vi "Write File.vi"(7 "Section":string, 8 "error in (no error)":errorcluster, 10 "Parameters":refnum<class "Parameter.lvclass">[](array[class]), 11 "Parameter INI File in":refnum<class "Parameter INI File.lvclass">) -> (0 "error out":errorcluster, 3 "Parameter INI File out":refnum<class "Parameter INI File.lvclass">)   [LabVIEW 2019, in "CD Parameter Manager API.lvlib" / "Parameter INI File.lvclass"]
uses:
  Parameter INI File.lvclass
  Parameter Class/Parameter.lvclass
  Parameter INI File.lvclass/Parameter INI File.ctl
  Double Parameter Class/Double Parameter.lvclass
  C:/Repositories/CSD_Custom_Device/CSD_Custom_Device/Source/Libraries/CD Parameter Manager API/Parameter Class/Parameter.lvclass
  Parameter Class/Parameter.lvclass/Parameter.ctl
  Double Parameter Class/Double Parameter.lvclass/Double Parameter.ctl
  Boolean Parameter Class/Boolean Parameter.lvclass
  Boolean Parameter Class/Boolean Parameter.lvclass/Boolean Parameter.ctl
  I32 Parameter Class/I32 Parameter.lvclass
  I32 Parameter Class/I32 Parameter.lvclass/I32 Parameter.ctl
  String Parameter Class/String Parameter.lvclass
  String Parameter Class/String Parameter.lvclass/String Parameter.ctl
  File Path Parameter Class/File Path Parameter.lvclass
  File Path Parameter Class/File Path Parameter.lvclass/File Path Parameter.ctl
  Parameter Class/Member Accessors/Read Control label.vi
  Double Parameter Class/Member Accessors/Read Value.vi
  Boolean Parameter Class/Member Accessors/Read Value.vi
  I32 Parameter Class/Member Accessors/Read Value.vi
  String Parameter Class/Member Accessors/Read Value.vi
  File Path Parameter Class/Member Accessors/Read Value.vi
  <vilib>/Utility/config.llb/Write Key (Double).vi
  <vilib>/Utility/config.llb/Write Key (Boolean).vi
  <vilib>/Utility/config.llb/Write Key (I32).vi
  <vilib>/Utility/config.llb/Write Key (String).vi
  <vilib>/Utility/config.llb/Write Key (Path).vi
  <vilib>/Utility/error.llb/Error Cluster From Error Code.vi
  <vilib>/ErrorRing/Error Ring.xnode
  <vilib>/Utility/config.llb/NI_LVConfig.lvlib
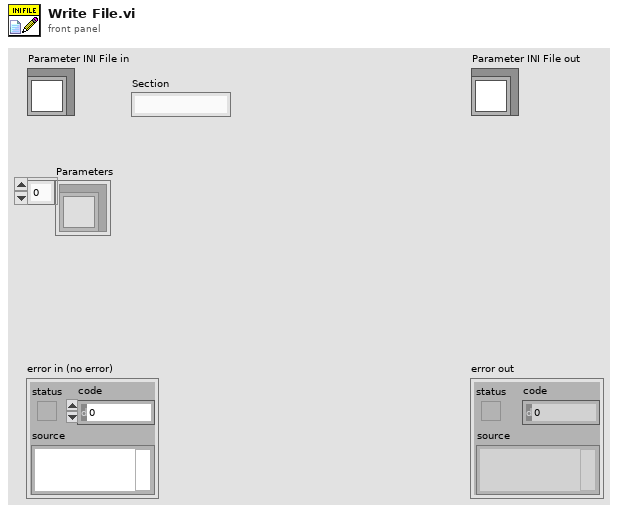
[diagram p1: front panel]
types:
  T1 = typedef "NI_LVConfig.lvlib/Config Data RefNum.ctl" = refnum<k1>
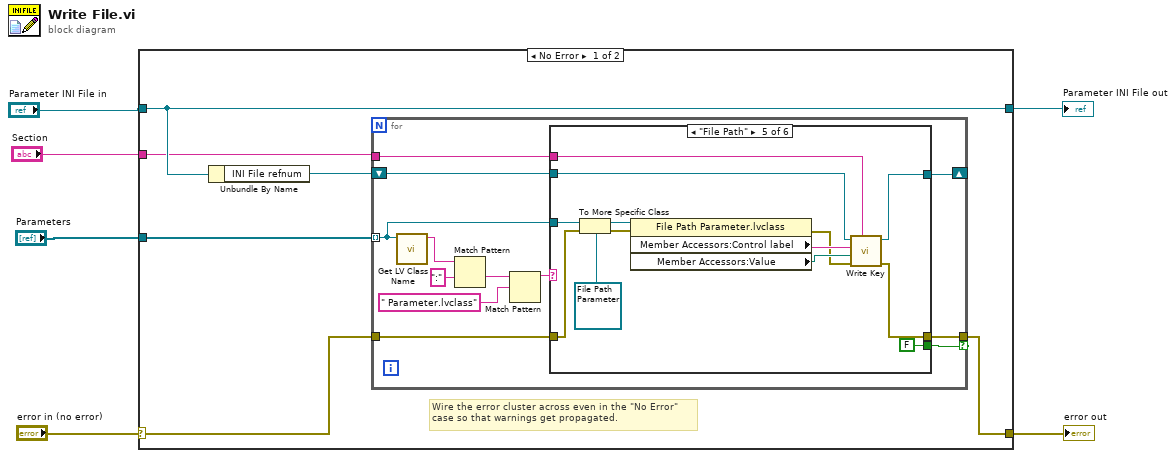
[diagram p0: block diagram]
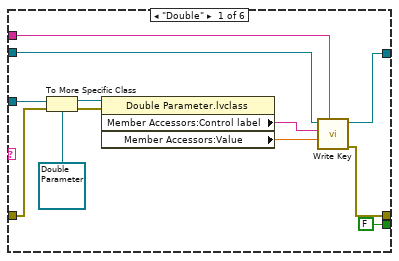
[diagram p2: hidden frame]
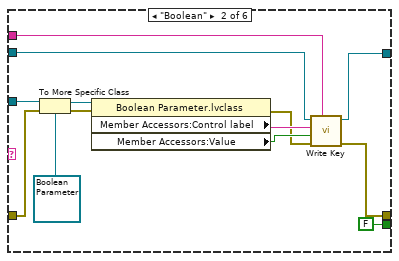
[diagram p3: hidden frame]
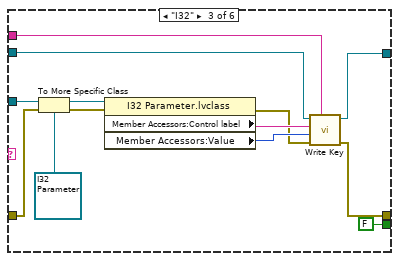
[diagram p4: hidden frame]
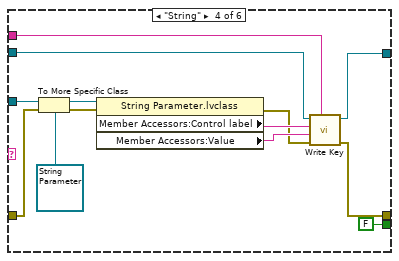
[diagram p5: hidden frame]
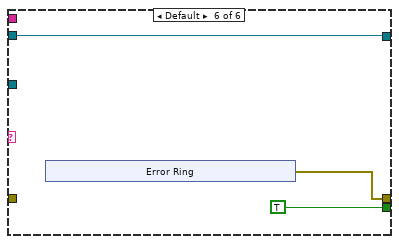
[diagram p6: hidden frame]
diagram:
  n1 = case shown="No Error" "error in (no error)" {
    selector: "error in (no error)" -> [w12 w98]
    tunnel: [w11 w98] -> w3
    tunnel: [w10 w97] -> w4
    tunnel: "Parameter INI File in" -> [w10 w97]
    tunnel: "Parameters" -> [w8 _]
    tunnel: "Section" -> [w7 _]
    frame No Error {
      # "Wire the error cluster across even in the \"No Error\"\ncase so that warnings get propagated."
      n2 = Unbundle By Name(w10) -> ("INI File refnum"=w9:T1)
      n3 = for {
        tunnel: w12 -> [w19]
        tunnel: [w14] -> w11 if=w15
        tunnel: w8 -> [w17] mode=indexing
        tunnel: w7 -> [w16]
        shift-right: [w13] -> _
        shift-left: w9 -> [w18]
        n4 = call <vilib>:"Get LV Class Name.vi"("object"=w17) -> ("class name"=w21:string)  [unwired: 9 in, 1 out]
        n5 = Match Pattern(string=w21, regular expression=":") -> (after substring=w23:string)  [unwired: 1 in, 3 out]
        n6 = Match Pattern(string=w23, regular expression=" Parameter.lvclass") -> (before substring=w20:string)  [unwired: 1 in, 3 out]
        n7 = case shown="\"File Path\"" w20 {
          tunnel: w19 -> [w32 w44 w57 w70 w83 _]
          tunnel: [w27 w43 w52 w66 w79 w90] -> w14
          tunnel: [FALSE ("found?") FALSE ("found?") FALSE ("found?") FALSE ("found?") FALSE ("found?") TRUE] -> w15
          tunnel: w18 -> [w28 w40 w55 w68 w81 w89]
          tunnel: w17 -> [w35 w45 w58 w71 w84 _]
          tunnel: w16 -> [w29 w41 w54 w67 w80 _]
          tunnel: [w25 w37 w50 w64 w77 w89] -> w13
          frame "Double" {
            n8 = To More Specific Class(target class=refnum<class "Double Parameter.lvclass"> refnum ("CD Parameter Manager API.lvlib:Double Parameter.lvclass"), reference=w35, error in=w32) -> (specific class reference=w34:refnum<class "Double Parameter.lvclass">, error out=w36:errorcluster)
            n9 = property class="Double Parameter.lvclass"(reference=w34, error in=w36) -> ("Member Accessors:Control label"=w30:string, "Member Accessors:Value"=w31:dbl)  [unwired: 2 out]
            n10 = call-poly <vilib>:"Write Key.vi"("section"=w29, "value"=w31, "key"=w30, "refnum"=w28) -> ("error out"=w27:errorcluster, "refnum out"=w25:T1)  [unwired: 5 in, 1 out]
          }
          frame "Boolean" {
            n11 = To More Specific Class(target class=refnum<class "Boolean Parameter.lvclass"> refnum ("CD Parameter Manager API.lvlib:Boolean Parameter.lvclass"), reference=w45, error in=w44) -> (specific class reference=w47:refnum<class "Boolean Parameter.lvclass">, error out=w48:errorcluster)
            n12 = property class="Boolean Parameter.lvclass"(reference=w47, error in=w48) -> (error out=w42:errorcluster, "Member Accessors:Control label"=w49:string, "Member Accessors:Value"=w46:bool)  [unwired: 1 out]
            n13 = call-poly <vilib>:"Write Key.vi"("section"=w41, "error in (no error)"=w42, "value"=w46, "key"=w49, "refnum"=w40) -> ("error out"=w43:errorcluster, "refnum out"=w37:T1)  [unwired: 4 in, 1 out]
          }
          frame "I32" {
            n14 = To More Specific Class(target class=refnum<class "I32 Parameter.lvclass"> refnum ("CD Parameter Manager API.lvlib:I32 Parameter.lvclass"), reference=w58, error in=w57) -> (specific class reference=w60:refnum<class "I32 Parameter.lvclass">, error out=w61:errorcluster)
            n15 = property class="I32 Parameter.lvclass"(reference=w60, error in=w61) -> (error out=w56:errorcluster, "Member Accessors:Control label"=w62:string, "Member Accessors:Value"=w59:i32)  [unwired: 1 out]
            n16 = call-poly <vilib>:"Write Key.vi"("section"=w54, "error in (no error)"=w56, "value"=w59, "key"=w62, "refnum"=w55) -> ("error out"=w52:errorcluster, "refnum out"=w50:T1)  [unwired: 4 in, 1 out]
          }
          frame "String" {
            n17 = To More Specific Class(target class=refnum<class "String Parameter.lvclass"> refnum ("CD Parameter Manager API.lvlib:String Parameter.lvclass"), reference=w71, error in=w70) -> (specific class reference=w73:refnum<class "String Parameter.lvclass">, error out=w74:errorcluster)
            n18 = property class="String Parameter.lvclass"(reference=w73, error in=w74) -> (error out=w69:errorcluster, "Member Accessors:Control label"=w75:string, "Member Accessors:Value"=w72:string)  [unwired: 1 out]
            n19 = call-poly <vilib>:"Write Key.vi"("section"=w67, "error in (no error)"=w69, "value"=w72, "key"=w75, "refnum"=w68) -> ("error out"=w66:errorcluster, "refnum out"=w64:T1)  [unwired: 4 in, 1 out]
          }
          frame "File Path" {
            n20 = To More Specific Class(target class=refnum<class "File Path Parameter.lvclass"> refnum ("CD Parameter Manager API.lvlib:File Path Parameter.lvclass"), reference=w84, error in=w83) -> (specific class reference=w86:refnum<class "File Path Parameter.lvclass">, error out=w87:errorcluster)
            n21 = property class="File Path Parameter.lvclass"(reference=w86, error in=w87) -> (error out=w82:errorcluster, "Member Accessors:Control label"=w88:string, "Member Accessors:Value"=w85:path)  [unwired: 1 out]
            n22 = call-poly <vilib>:"Write Key.vi"("section"=w80, "error in (no error)"=w82, "value"=w85, "key"=w88, "refnum"=w81) -> ("error out"=w79:errorcluster, "refnum out"=w77:T1)  [unwired: 4 in, 1 out]
          }
          frame Default {
            n23 = xnode "Error Ring"() -> ("error out"=w90:errorcluster)
          }
        }
      }
    }
    frame Error {
    }
  }
  "error out" <- w3
  "Parameter INI File out" <- w4
